vi "Delete AIs RT FIFO.vi"(8 "error in":errorcluster, 11 "AIs RT FIFO":refnum<k33>) -> (0 "error out":errorcluster)   [LabVIEW 2021, in "RT Main.lvlib"]
uses:
  RT Main.lvlib
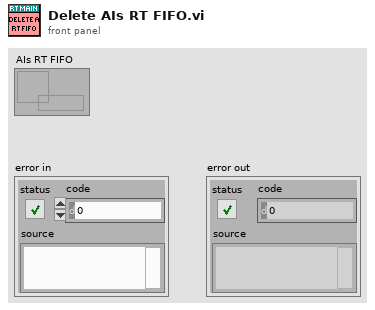
[diagram p1: front panel]
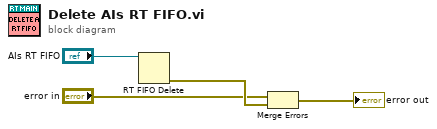
[diagram p0: block diagram]
diagram:
  n1 = RT FIFO Delete(0:"AIs RT FIFO") -> (11:w4:errorcluster)  [unwired: 2 in]
  n2 = Merge Errors("error in", w4) -> (→"error out":errorcluster)
